vi "Controller Generate PID Filter Coefficients.vi"(9 "Period":dbl, 10 "Derivative Time":dbl, 11 "Integral Time":dbl) -> (2 "Scaling Gain":dbl, 3 "PS Filter Coefficients":dbl[](array[numeric]))   [LabVIEW 2011, in "Controller VIs.lvlib"]
uses:
  Controller VIs.lvlib
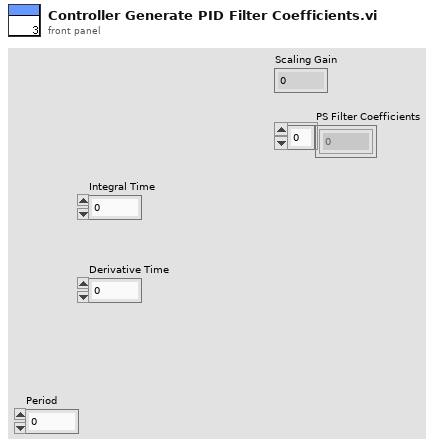
[diagram p1: front panel]
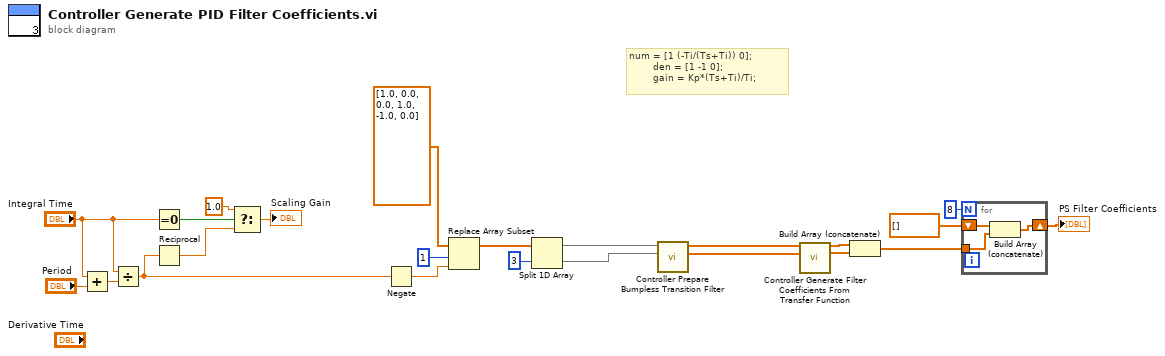
[diagram p0: block diagram]
diagram:
  # "num = [1 (-Ti/(Ts+Ti)) 0];\n        den = [1 -1 0];\n        gain = Kp*(Ts+Ti)/Ti;"
  n1 = Add(x="Integral Time", y="Period") -> (x+y=w11:dbl)
  n2 = Divide(x="Integral Time", y=w11) -> (x/y=w12:dbl)
  n3 = Equal To 0?(x="Integral Time") -> (x = 0?=w17:bool)
  n4 = Reciprocal(x=w12) -> (1/x=w14:dbl)
  n5 = Select(t=1.0, s=w17, f=w14) -> (s? t:f=→"Scaling Gain":dbl)
  n6 = Negate(x=w12) -> (-x=w13:dbl)
  n7 = Replace Array Subset(array=dbl[] [1.0, 0.0, 0.0, 1.0, -1.0, 0.0] ("coeffs"), new element=w13, index=1) -> (w19:dbl[])
  n8 = Split 1D Array(array=w19, index=3) -> (first subarray=w2:dbl[], second subarray=w22:dbl[])
  n9 = call "Controller Prepare Bumpless Transition Filter.vi"("den in"=w22, "num in"=w2) -> ("den out"=w1:dbl[], "num out"=w23:dbl[])  [unwired: 7 in, 1 out]
  n10 = call "Controller Generate Filter Coefficients From Transfer Function.vi"("numerator"=w23, "denominator"=w1) -> ("coeff b"=w4:dbl[], "coeff a"=w3:dbl[])  [unwired: 11 in, 1 out]
  n11 = Build Array (concatenate)(w4, w3) -> (w20:dbl[])
  n12 = for {
    N: 8 -> [_]
    tunnel: w20 -> [w25]
    shift-right: [w24] -> w9
    shift-left: dbl[] [] ("Array") -> [w26]
    n13 = Build Array (concatenate)(w26, w25) -> (w24:dbl[])
  }
  "PS Filter Coefficients" <- w9
